vi "Tree_Set position based on value.vi"(8 "error in (no error)":errorcluster, 10 "Selected Row":i32=-1, 11 "Tree Ref":refnum<vi>) -> (0 "error out":errorcluster, 3 "Tree Ref":refnum<vi>)   [LabVIEW 2023]
doc: "Sets position of the current tree value to fall within the view range of the list box. Since tree may also be multi-select, you can instead pass in the index of the selected row to scroll to.\n\nThis works with single-select and multi-select trees, as long as they have array data types"
uses:
  <vilib>/Utility/miscctls.llb/LVNodeAndColumnTypeDef.ctl
panel:
  out "Value":i32
  out "number of items":i32
  in  "Tree":string[](tree)
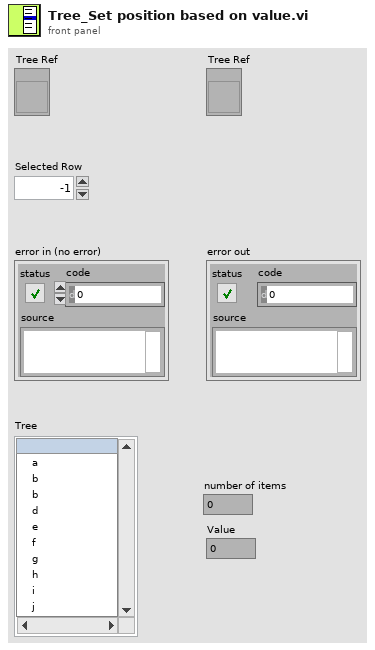
[diagram p1: front panel]
types:
  T1 = typedef "LVNodeAndColumnTypeDef.ctl" = cluster{"Node":string, "Column":i32}
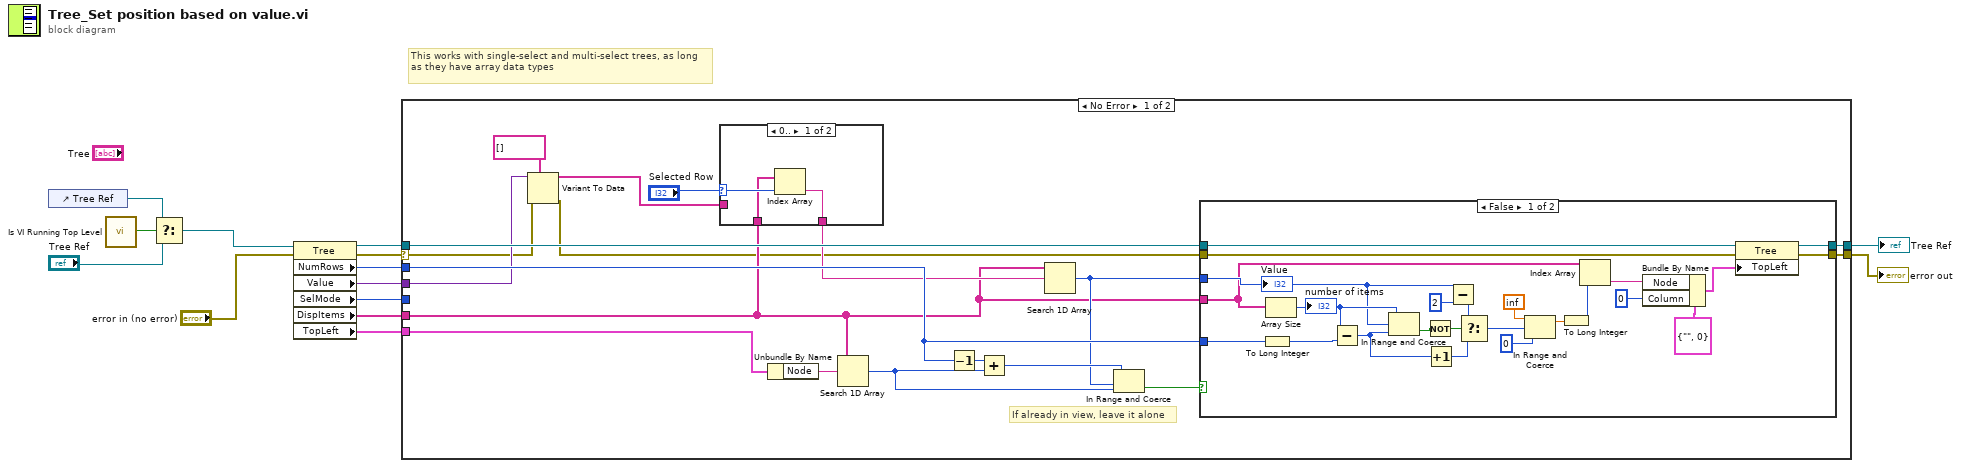
[diagram p0: block diagram]
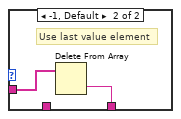
[diagram p2: hidden frame]
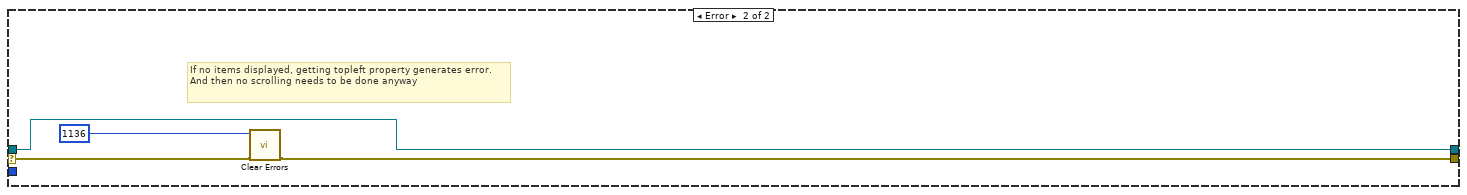
[diagram p4: hidden frame]
diagram:
  # "This works with single-select and multi-select trees, as long as they have array data types"
  n1 = control-ref of="Tree Ref"() -> (w9:refnum<vi>)
  n2 = call "Is VI Running Top Level.vi"() -> ("Top Level?"=w13:bool)  [unwired: 5 in]
  n3 = Select(t=w9, s=w13, f="Tree Ref") -> (s? t:f=w12:refnum<vi>)
  n4 = property class="Tree"(reference=w12, error in="error in (no error)") -> (reference out=w14:refnum<vi>, error out=w2:errorcluster, "NumRows"=w10:u32, "Value"=w3:variant, "SelMode"=w1:i32, "DispItems"=w4:string[], "TopLeft"=w8:T1)
  n5 = case shown="No Error" w2 {
    selector: w2 -> [w16 w68]
    tunnel: w14 -> [w33 w66]
    tunnel: w10 -> [w32 _]
    tunnel: w8 -> [w31 _]
    tunnel: [w29 w65] -> w7
    tunnel: [w23 w66] -> w6
    tunnel: w4 -> [w20 _]
    tunnel: w3 -> [w19 _]
    tunnel: w1 -> [_ _]
    frame No Error {
      # "If already in view, leave it alone"
      n6 = Variant To Data(error in=w16, type=string[] [], Variant=w19) -> (data=w18:string[], error out=w17:errorcluster)
      n7 = case shown="0.." "Selected Row" {
        selector: "Selected Row" -> [w36 _]
        tunnel: [w35 w38] -> w22
        tunnel: w20 -> [w34 _]
        tunnel: w18 -> [_ w37]
        frame 0.. {
          n8 = Index Array(array=w34, index=w36) -> (element=w35:string)
        }
        frame -1, Default {
          # "Use last value element"
          n9 = Delete From Array(array=w37) -> (deleted portion=w38:string)  [unwired: 2 in, 1 out]
        }
      }
      n10 = Unbundle By Name(w31) -> ("Node"=w30:string)
      n11 = Search 1D Array(1D array=w20, element=w30) -> (index of element=w24:i32)  [unwired: 1 in]
      n12 = Decrement(x=w32) -> (x-1=w27:u32)
      n13 = Add(x=w27, y=w24) -> (x+y=w26:u32)
      n14 = Search 1D Array(1D array=w20, element=w22) -> (index of element=w25:i32)  [unwired: 1 in]
      n15 = In Range and Coerce(upper limit=w26, x=w25, lower limit=w24) -> (In Range?=w28:bool)  [unwired: 1 out]
      n16 = case shown="False" w28 {
        tunnel: w20 -> [w44 _]
        tunnel: w33 -> [w62 w64]
        tunnel: w17 -> [w49 w63]
        tunnel: [w48 w64] -> w23
        tunnel: [w47 w63] -> w29
        tunnel: w25 -> [w46 _]
        tunnel: w32 -> [w45 _]
        frame False {
          n17 = To Long Integer(number=w45) -> (32bit integer=w51:i32)
          n18 = Array Size(array=w44) -> (size(s)=w61:i32)
          "number of items" <- w61
          n19 = Subtract(x=w61, y=w51) -> (x-y=w57:i32)
          n20 = In Range and Coerce(upper limit=w61, x=w46, lower limit=w57) -> (In Range?=w59:bool)  [unwired: 1 out]
          n21 = Not(x=w59) -> (.not. x?=w58:bool)
          n22 = Increment(x=w57) -> (x+1=w56:i32)
          n23 = Subtract(x=w46, y=2) -> (x-y=w50:i32)
          n24 = Select(t=w50, s=w58, f=w56) -> (s? t:f=w53:i32)
          n25 = In Range and Coerce(upper limit=inf, x=w53, lower limit=u32 0 ("upper limit")) -> (coerced(x)=w52:dbl)  [unwired: 1 out]
          n26 = To Long Integer(number=w52) -> (32bit integer=w43:i32)
          n27 = Index Array(array=w44, index=w43) -> (element=w39:string)
          n28 = Bundle By Name(cluster=T1 {"Node"="", "Column"=0} ("Top Left Visible Cell"), "Node"=w39, "Column"=0) -> (w42:T1)
          n29 = property class="Tree"(reference=w62, error in=w49, "TopLeft"=w42) -> (reference out=w48:refnum<vi>, error out=w47:errorcluster)
          "Value" <- w46
        }
        frame True {
        }
      }
    }
    frame Error {
      # "If no items displayed, getting topleft property generates error. And then no scrolling needs to be done anyway"
      n30 = call <vilib>:"Clear Errors.vi"("error in (no error)"=w68, "specific error code to clear (0: all)"=1136) -> ("error out"=w65:errorcluster)  [unwired: 4 in, 1 out]
    }
  }
  "Tree Ref" <- w6
  "error out" <- w7
